vi "Replace_Element.vi"(2 "error in (no error)":errorcluster, 3 "Numeric":i32, 4 "cluster":cluster{"Test Name":string, "File Path":path}, 5 "Queue in":refnum<queue>) -> (0 "error out":errorcluster, 1 "Queue out":refnum<queue>)   [LabVIEW 2018]
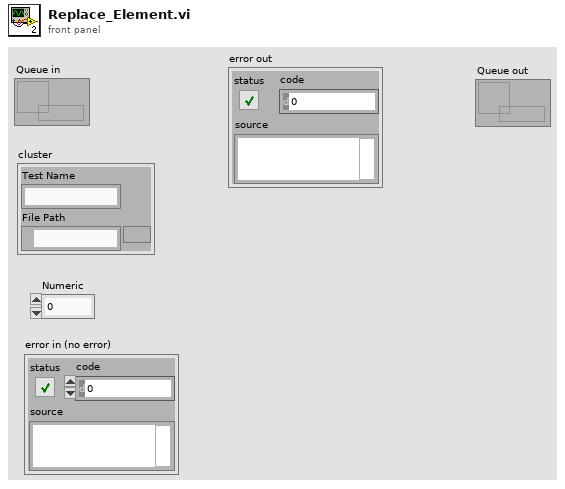
[diagram p1: front panel]
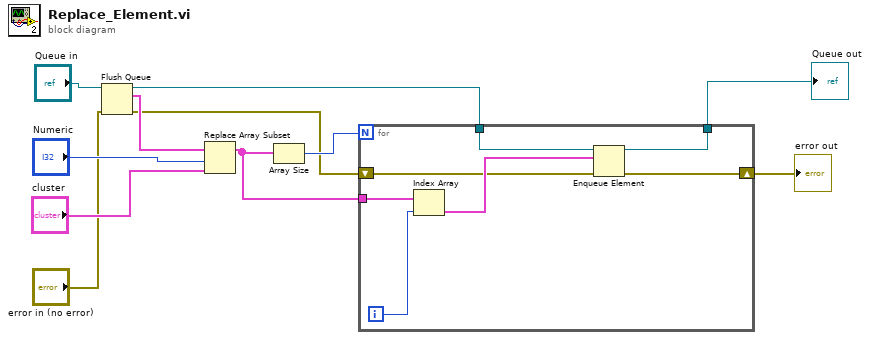
[diagram p0: block diagram]
diagram:
  n1 = Flush Queue(queue="Queue in", error in (no error)="error in (no error)") -> (queue out=w6:refnum<queue>, remaining elements=w10:cluster{"Test Name":string, "File Path":path}[], error out=w1:errorcluster)
  n2 = Replace Array Subset(array=w10, new element="cluster", index="Numeric") -> (w5:cluster{"Test Name":string, "File Path":path}[])
  n3 = Array Size(array=w5) -> (size(s)=w7:i32)
  n4 = for {
    N: w7 -> [_]
    tunnel: w6 -> [w18]
    tunnel: w5 -> [w17]
    tunnel: [w14] -> w3
    shift-right: [w13] -> w2
    shift-left: w1 -> [w12]
    i -> [w16]
    n5 = Index Array(array=w17, index=w16) -> (element=w15:cluster{"Test Name":string, "File Path":path})
    n6 = Enqueue Element(queue=w18, element=w15, error in (no error)=w12) -> (queue out=w14:refnum<queue>, error out=w13:errorcluster)  [unwired: 1 in, 1 out]
  }
  "Queue out" <- w3
  "error out" <- w2
